vi "MFLI Create a and set module.vi"(8 "error in (no error)":errorcluster, 10 "module Id":T2 items=["sweep", "scopeModule", "dataAcquisitionModule", "pidAdvisor", "awgModule", "impedanceModule", "multiDeviceSyncModule", "zoomFFT", "trigger", "deviceSettings", "record", "precompensationAdvisor"], 11 "Lock-in Handle":T1 {"Handle" format="0x%08x"; "Conn" format="0x%08x"}) -> (0 "Error Out":errorcluster, 2 "ModHandle Out":T3 {"ModHandle" format="0x%08x"; "Conn" format="0x%08x"}, 3 "Lock-in Handle out":T1 {"Handle" format="0x%08x"; "Conn" format="0x%08x"})   [LabVIEW 2022 SP3, in "Lock-in module.lvlib"]
uses:
  Lock-in module.lvlib
  <instrlib>/Zurich Instruments LabOne/Public/Modules/ziTypeModHandle.ctl
  <instrlib>/Zurich Instruments LabOne/Public/Modules/ziTypeModEnum.ctl
  <instrlib>/Zurich Instruments LabOne/Public/ziTypeHandle.ctl
  <instrlib>/Zurich Instruments LabOne/Public/Modules/ziModSetValueDoubleArray.vi
  <instrlib>/Zurich Instruments LabOne/Public/Configure/ziSetValueDoubleArray.vi
  <instrlib>/Zurich Instruments LabOne/Public/Modules/ziModSetValueBinary.vi
  <instrlib>/Zurich Instruments LabOne/Zurich Instruments LabOne.lvlib
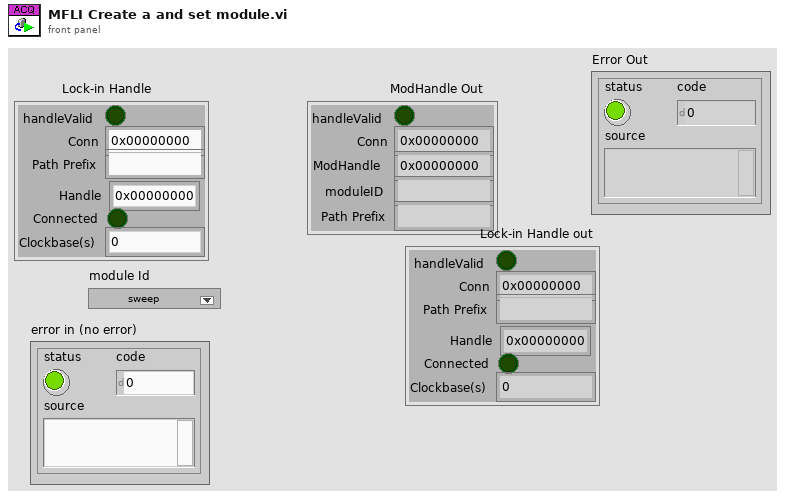
[diagram p1: front panel]
types:
  T1 = typedef "Zurich Instruments LabOne.lvlib/ziTypeHandle.ctl" = cluster{"handleValid":bool, "Conn":u64, "Path Prefix":string, "Handle":u64, "Connected":bool, "Clockbase(s)":dbl}
  T2 = typedef "Zurich Instruments LabOne.lvlib/ziTypeModEnum.ctl" = u16
  T3 = typedef "Zurich Instruments LabOne.lvlib/ziTypeModHandle.ctl" = cluster{"handleValid":bool, "Conn":u64, "ModHandle":u64, "moduleID":string, "Path Prefix":string}
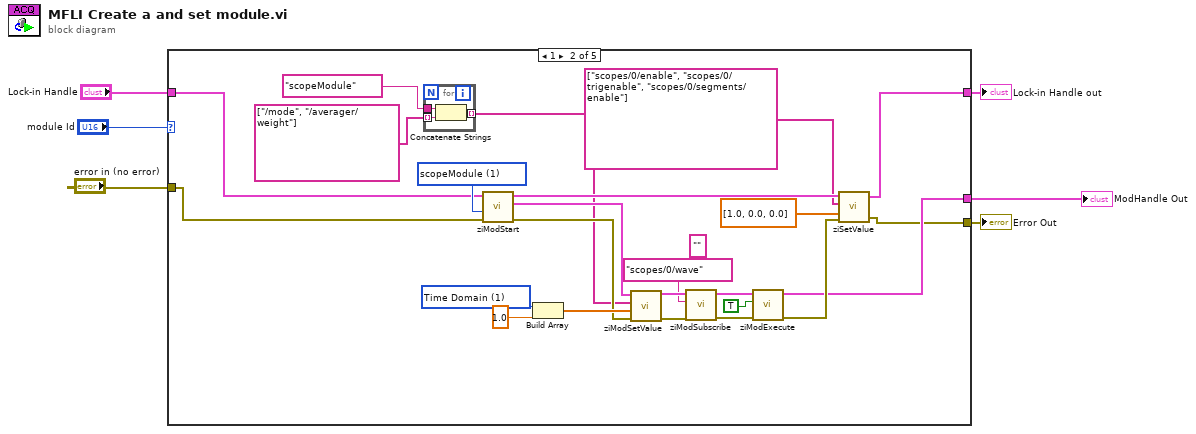
[diagram p0: block diagram]
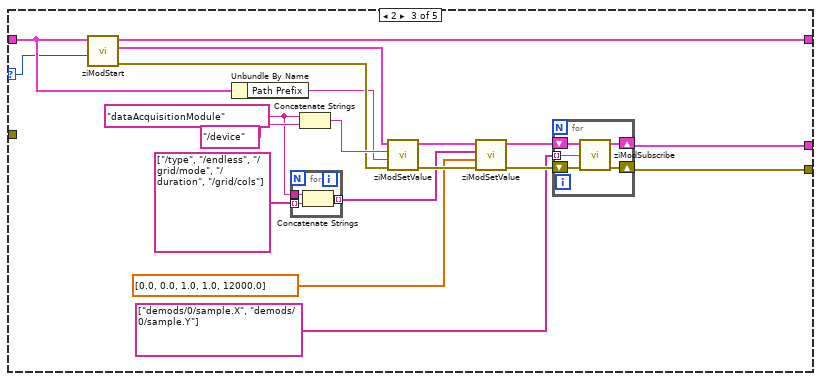
[diagram p3: hidden frame]
diagram:
  n1 = case shown="1" "module Id" {
    selector: "module Id" -> [_ _ w35 _ _]
    tunnel: [_ w8 w53 _ _] -> w2
    tunnel: [_ w14 w52 _ _] -> w5
    tunnel: "Lock-in Handle" -> [w7 w13 w37 w62 w63]
    tunnel: [w7 w15 w39 w62 w63] -> w1
    tunnel: "error in (no error)" -> [_ w9 _ _ _]
    frame 0, Default {
    }
    frame 1 {
      w20 = u16 1 items=["Time Domain"=1, "Freq Domain FFT"=3] ("mode")
      w18 = T2 1 items=["sweep", "scopeModule", "dataAcquisitionModule", "pidAdvisor", "awgModule", "impedanceModule", "multiDeviceSyncModule", "zoomFFT", "trigger", "deviceSettings", "record"] ("module Id")
      (unwired) ""
      n2 = for {
        tunnel: string[] ["/mode", "/averager/weight"] -> [w34] mode=indexing
        tunnel: "scopeModule" -> [w33]
        tunnel: [w32] -> w10 mode=indexing
        n3 = Concatenate Strings(w33, w34) -> (w32:string)
      }
      n4 = call <instrlib>:"ziModStart.vi"("Error In"=w9, "module Id"=w18, "Handle In"=w13) -> ("Error Out"=w29:errorcluster, "ModHandle Out"=w28:T3, "Handle Out"=w30:T1)  [unwired: 6 in]
      n5 = Build Array(w20, 1.0 ("averagerweight")) -> (w31:dbl[])
      n6 = call-poly <instrlib>:"ziModSetValue.vi"("Error In"=w29, "Values"=w31, "Paths"=w10, "ModHandle In"=w28) -> ("Error Out"=w24:errorcluster, "ModHandle Out"=w25:T3)  [unwired: 6 in]
      n7 = call <instrlib>:"ziModSubscribe.vi"("Error In"=w24, "Path"="scopes/0/wave", "ModHandle In"=w25) -> ("Error Out"=w26:errorcluster, "ModHandle Out"=w27:T3)  [unwired: 6 in]
      n8 = call <instrlib>:"ziModExecute.vi"("Error In"=w26, "Modal (F)"=TRUE ("Modal"), "ziModHandle In"=w27) -> ("Error Out"=w23:errorcluster, "ziModHandle Out"=w14:T3)  [unwired: 5 in, 1 out]
      n9 = call-poly <instrlib>:"ziSetValue.vi"("Error In"=w23, "Values"=dbl[] [1.0, 0.0, 0.0] ("Value"), "Paths"=string[] ["scopes/0/enable", "scopes/0/trigenable", "scopes/0/segments/enable"], "Handle In"=w30) -> ("Error Out"=w8:errorcluster, "Handle Out"=w15:T1)  [unwired: 1 in]
    }
    frame 2 {
      w42 = "dataAcquisitionModule"
      n10 = call <instrlib>:"ziModStart.vi"("module Id"=w35, "Handle In"=w37) -> ("Error Out"=w38:errorcluster, "ModHandle Out"=w40:T3, "Handle Out"=w39:T1)  [unwired: 7 in]
      n11 = Unbundle By Name(w37) -> ("Path Prefix"=w36:string)
      n12 = for {
        tunnel: string[] ["/type", "/endless", "/grid/mode", "/duration", "/grid/cols"] -> [w56] mode=indexing
        tunnel: w42 -> [w55]
        tunnel: [w54] -> w41 mode=indexing
        n13 = Concatenate Strings(w55, w56) -> (w54:string)
      }
      n14 = Concatenate Strings(w42, "/device") -> (w44:string)
      n15 = call-poly <instrlib>:"ziModSetValue.vi"("Error In"=w38, "Data"=w36, "Path"=w44, "ModHandle In"=w40) -> ("Error Out"=w48:errorcluster, "ModHandle Out"=w47:T3)  [unwired: 6 in]
      n16 = call-poly <instrlib>:"ziModSetValue.vi"("Error In"=w48, "Values"=dbl[] [0.0, 0.0, 1.0, 1.0, 12000.0], "Paths"=w41, "ModHandle In"=w47) -> ("Error Out"=w50:errorcluster, "ModHandle Out"=w51:T3)  [unwired: 6 in]
      n17 = for {
        shift-right: [w61] -> w52
        shift-left: w51 -> [w58]
        tunnel: string[] ["demods/0/sample.X", "demods/0/sample.Y"] ("subscribe") -> [w60] mode=indexing
        shift-right: [w57] -> w53
        shift-left: w50 -> [w59]
        n18 = call <instrlib>:"ziModSubscribe.vi"("Error In"=w59, "Path"=w60, "ModHandle In"=w58) -> ("Error Out"=w57:errorcluster, "ModHandle Out"=w61:T3)  [unwired: 6 in]
      }
    }
    frame 3 {
    }
    frame 4 {
    }
  }
  "ModHandle Out" <- w5
  "Error Out" <- w2
  "Lock-in Handle out" <- w1
